vi "solar_tcp Bits Get.vi"(9 "Bit Size (0..64)":i32, 10 "Bit Offset (0)":i32, 11 "Data":string) -> (1 "Value as I32":i32, 2 "Value (Binary) [Byte aligned]":string, 3 "dup Data":string)   [LabVIEW 2018]
doc: "This returns the byte aligned value from <b>Data</b> specified by <b>Bit Offset</b> and <b>Bit Size</b>. Note: This only supports up to 64 bits."
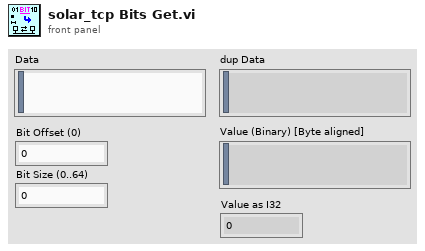
[diagram p1: front panel]
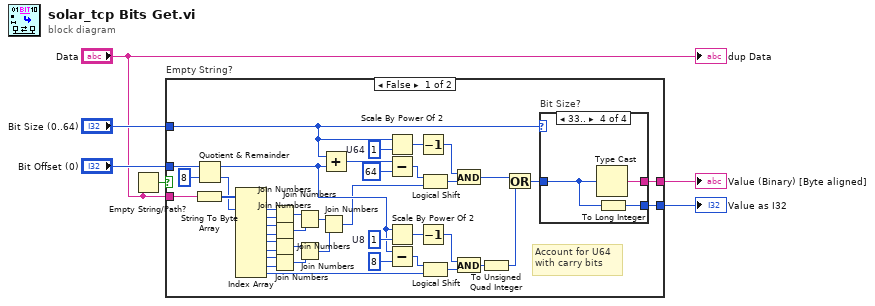
[diagram p0: block diagram]
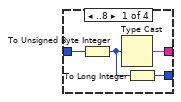
[diagram p2: hidden frame]
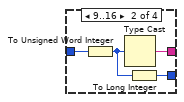
[diagram p3: hidden frame]
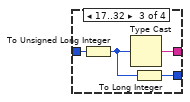
[diagram p4: hidden frame]
diagram:
  n1 = Empty String/Path?(string/path="Data") -> (empty?=w1:bool)
  n2 = case "Empty String?" shown="False" w1 {
    tunnel: "Data" -> [w36 _]
    tunnel: [w48 _] -> w6
    tunnel: [w47 _] -> w5
    tunnel: "Bit Offset (0)" -> [w46 _]
    tunnel: "Bit Size (0..64)" -> [w45 _]
    frame False {
      w19 = u8 1  # U8
      w40 = u64 1  # U64
      # "Account for U64\nwith carry bits"
      n3 = String To Byte Array(string=w36) -> (unsigned byte array=w35:u8[])
      n4 = Quotient & Remainder(x=w46, y=8) -> (x-y*floor(x/y)=w18:i32, floor(x/y)=w8:i32)
      n5 = Index Array(array=w35, index #1=w8) -> (element #1=w34:u8, element #2=w33:u8, element #3=w32:u8, element #4=w31:u8, element #5=w30:u8, element #6=w29:u8, element #7=w28:u8, element #8=w27:u8, element #9=w14:u8)  [unwired: 8 in]
      n6 = Join Numbers(hi=w34, lo=w33) -> ((hi.lo)=w26:u16)
      n7 = Join Numbers(hi=w32, lo=w31) -> ((hi.lo)=w24:u16)
      n8 = Join Numbers(hi=w30, lo=w29) -> ((hi.lo)=w25:u16)
      n9 = Join Numbers(hi=w28, lo=w27) -> ((hi.lo)=w23:u16)
      n10 = Join Numbers(hi=w26, lo=w24) -> ((hi.lo)=w22:u32)
      n11 = Join Numbers(hi=w25, lo=w23) -> ((hi.lo)=w21:u32)
      n12 = Join Numbers(hi=w22, lo=w21) -> ((hi.lo)=w7:u64)
      n13 = Add(x=w45, y=w18) -> (x+y=w43:i32)
      n14 = Scale By Power Of 2(n=w45, x=w40) -> (x*2^n=w39:u64)
      n15 = Subtract(x=w43, y=64) -> (x-y=w37:i32)
      n16 = Scale By Power Of 2(n=w18, x=w19) -> (x*2^n=w20:u8)
      n17 = Subtract(x=w18, y=8) -> (x-y=w15:i32)
      n18 = Decrement(x=w39) -> (x-1=w38:u64)
      n19 = Decrement(x=w20) -> (x-1=w16:u8)
      n20 = Logical Shift(y=w37, x=w7) -> (x << y=w41:u64)
      n21 = Logical Shift(y=w15, x=w14) -> (x << y=w13:u8)
      n22 = And(x=w38, y=w41) -> (x .and. y?=w10:u64)
      n23 = And(x=w16, y=w13) -> (x .and. y?=w12:u8)
      n24 = To Unsigned Quad Integer(1:w12) -> (0:w11:u64)
      n25 = Or(x=w10, y=w11) -> (x .or. y?=w9:u64)
      n26 = case "Bit Size?" shown="33.." w45 {
        tunnel: [w52 w56 w60 w63] -> w48
        tunnel: w9 -> [w51 w55 w59 w62]
        tunnel: [w49 w53 w57 w61] -> w47
        frame ..8 {
          n27 = To Unsigned Byte Integer(number=w51) -> (unsigned 8bit integer=w50:u8)
          n28 = Type Cast(x=w50) -> (*(type *) &x=w52:string)  [unwired: 1 in]
          n29 = To Long Integer(number=w50) -> (32bit integer=w49:i32)
        }
        frame 9..16 {
          n30 = To Unsigned Word Integer(number=w55) -> (unsigned 16bit integer=w54:u16)
          n31 = Type Cast(x=w54) -> (*(type *) &x=w56:string)  [unwired: 1 in]
          n32 = To Long Integer(number=w54) -> (32bit integer=w53:i32)
        }
        frame 17..32 {
          n33 = To Unsigned Long Integer(number=w59) -> (unsigned 32bit integer=w58:u32)
          n34 = Type Cast(x=w58) -> (*(type *) &x=w60:string)  [unwired: 1 in]
          n35 = To Long Integer(number=w58) -> (32bit integer=w57:i32)
        }
        frame 33.. {
          n36 = Type Cast(x=w62) -> (*(type *) &x=w63:string)  [unwired: 1 in]
          n37 = To Long Integer(number=w62) -> (32bit integer=w61:i32)
        }
      }
    }
    frame True {
    }
  }
  "Value (Binary) [Byte aligned]" <- w6
  "Value as I32" <- w5
  "dup Data" <- "Data"
